vi "errorToString.vi"(8 "error in (no error)":errorcluster, 11 "errorCode":i32) -> (0 "error out":errorcluster, 3 "errorMsg":string)   [LabVIEW 2011, in "sbgLabView.lvlib"]
uses:
  sbgLabView.lvlib
  sbgMatLab.dll
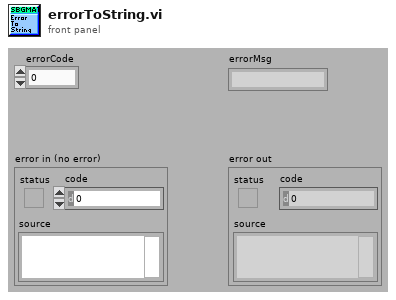
[diagram p1: front panel]
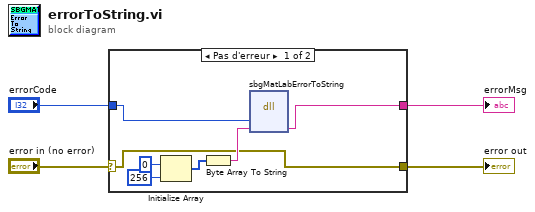
[diagram p0: block diagram]
diagram:
  n1 = case shown="Pas d'erreur" "error in (no error)" {
    selector: "error in (no error)" -> [w5 w12]
    tunnel: [w5 w12] -> w3
    tunnel: "errorCode" -> [w11 _]
    tunnel: [w6 _] -> w1
    frame No Error {
      n2 = Initialize Array(u8 0 ("element"), 256 ("dimension size")) -> (w10:u8[])
      n3 = Byte Array To String(unsigned byte array=w10) -> (string=w9:string)
      n4 = dll-call lib="C:/SBG-Systems/remote/projects/software/projects/labviewExample/sbgLabView/sbgMatLab.*" fn="sbgMatLabErrorToString"("errorCode"=w11, "errorMsg"=w9) -> ("errorMsg"=w6:string)  [unwired: 5 in, 2 out]
    }
    frame Error {
    }
  }
  "errorMsg" <- w1
  "error out" <- w3
